vi "Read.vi"(0 "session in":T1[](array[typedef]) {"rx baseband session"."3630 session"."Address Space" items=["VXI/VME A16"=1, "VXI/VME A24"=2, "VXI/VME A32"=3, "VXI/VME A64"=4, "PXI Memory Allocations"=9, "PXI Configuration"=10, "PXI BAR0"=11, "PXI BAR1"=12, "PXI BAR2"=13, "PXI BAR3"=14, "PXI BAR4"=15, "PXI BAR5"=16]; "tx baseband session"."3610 session"."Address Space" items=["VXI/VME A16"=1, "VXI/VME A24"=2, "VXI/VME A32"=3, "VXI/VME A64"=4, "PXI Memory Allocations"=9, "PXI Configuration"=10, "PXI BAR0"=11, "PXI BAR1"=12, "PXI BAR2"=13, "PXI BAR3"=14, "PXI BAR4"=15, "PXI BAR5"=16]}, 7 "number of samples":u32=8192, 9 "master device index":i32, 11 "error in":errorcluster, 12 "Timeout (ms)":i32=5000) -> (4 "session out":T1[](array[typedef]) {"rx baseband session"."3630 session"."Address Space" items=["VXI/VME A16"=1, "VXI/VME A24"=2, "VXI/VME A32"=3, "VXI/VME A64"=4, "PXI Memory Allocations"=9, "PXI Configuration"=10, "PXI BAR0"=11, "PXI BAR1"=12, "PXI BAR2"=13, "PXI BAR3"=14, "PXI BAR4"=15, "PXI BAR5"=16]; "tx baseband session"."3610 session"."Address Space" items=["VXI/VME A16"=1, "VXI/VME A24"=2, "VXI/VME A32"=3, "VXI/VME A64"=4, "PXI Memory Allocations"=9, "PXI Configuration"=10, "PXI BAR0"=11, "PXI BAR1"=12, "PXI BAR2"=13, "PXI BAR3"=14, "PXI BAR4"=15, "PXI BAR5"=16]}, 8 "data [channel]":cluster{"data":cdb[]}[](array[cluster]), 15 "error out":errorcluster)   [LabVIEW 2019, in "mmWave HW Control.lvlib"]
uses:
  mmWave HW Control.lvlib
  Low-level/TypeDefs/Session.ctl
  <instrlib>/niMmWave/ni3620/Config/v1/Host/Public/High-Level/niMmWave Session.ctl
  <instrlib>/_niInstr/Register Bus/v0/Host/Public/Register Bus Session.ctl
  <instrlib>/_niInstr/Register Bus/v0/Host/Private/Session Data.ctl
  <instrlib>/niMmWave/ni3620/Config/v1/Host/Public/Typedefs/Board Information.ctl
  <instrlib>/niMmWave/ni3620/Config/v1/Host/Public/Typedefs/Hardware Revision.ctl
  <instrlib>/niMmWave/ni3620/Config/v1/Host/Public/Typedefs/Gain Mapping.ctl
  <instrlib>/niMmWave/ni3620/Config/v1/Host/Public/Typedefs/Correction Data.ctl
  <instrlib>/niMmWave/ni3620/Config/v1/Host/Public/Typedefs/Opera Characterization.ctl
  <instrlib>/niMmWave/ni3620/Config/v1/Host/Public/Corrections/Typedefs/Opera Characterization Main Header.ctl
  <instrlib>/niMmWave/ni3620/Config/v1/Host/Public/Corrections/Typedefs/Opera IF Board Information.ctl
  <instrlib>/niMmWave/ni3620/Config/v1/Host/Public/Corrections/Typedefs/Opera Characterization Instance Header.ctl
  <instrlib>/niMmWave/ni3620/Config/v1/Host/Public/Corrections/Typedefs/Opera Characterization Device Data Header.ctl
  <instrlib>/niMmWave/ni3620/Config/v1/Host/Public/Corrections/Typedefs/Opera LO Characterization Data Header.ctl
  <instrlib>/niMmWave/ni3620/Config/v1/Host/Public/Corrections/Typedefs/Opera IF Board Characterization Data Header.ctl
  <instrlib>/niMmWave/ni3620/Config/v1/Host/Public/Corrections/Typedefs/Opera Characterization Device Data.ctl
  <instrlib>/niMmWave/ni3620/Config/v1/Host/Public/Corrections/Typedefs/Opera LO2 Board Characterization Data.ctl
  <instrlib>/niMmWave/ni3620/Config/v1/Host/Public/Corrections/Typedefs/Opera LO Characterization Data.ctl
  <instrlib>/niMmWave/ni3620/Config/v1/Host/Public/Corrections/Typedefs/Opera IF Board Characterization Data.ctl
  <instrlib>/niMmWave/ni3620/Config/v1/Host/Public/Corrections/Typedefs/Opera IQ Impairment Data.ctl
  <instrlib>/niMmWave/ni3620/Config/v1/Host/Public/Typedefs/mmWave Adapter Session Data.ctl
  <instrlib>/niMmWave/ni3620/Config/v1/Host/Public/Typedefs/mmWave Adapter Data.ctl
  <instrlib>/niMmWave/ni3620/Config/v1/Host/Public/Typedefs/mmWave Adapter 2.ctl
  <instrlib>/niMmWave/ni3620/Config/v1/Shared/Typedefs/Subsystem ID.ctl
  <instrlib>/niMmWave/ni3620/Config/v1/Host/Public/Typedefs/mmWave Adapter Channel Information.ctl
  <instrlib>/niMmWave/ni3620/Config/v1/Host/Public/Typedefs/Temperature Coefficients.ctl
  <instrlib>/niMmWave/ni3620/Config/v1/Host/Public/Typedefs/mmWave Characterization.ctl
  <instrlib>/niMmWave/ni3620/Config/v1/Host/Public/Corrections/Typedefs/mmWave Characterization Main Header.ctl
  <instrlib>/niMmWave/ni3620/Config/v1/Host/Public/Corrections/Typedefs/mmWave Characterization Instance Header.ctl
  <instrlib>/niMmWave/ni3620/Config/v1/Host/Public/Typedefs/Session Cache.ctl
  <instrlib>/niMmWave/ni3620/Config/v1/Host/Public/Typedefs/LO2 settings cache.ctl
  <instrlib>/niMmWave/ni3620/Config/v1/Host/Public/Typedefs/LO2 source.ctl
  <instrlib>/niMmWave/ni3620/Config/v1/Host/Public/Typedefs/Desired and Coerced.ctl
  <instrlib>/niMmWave/ni3620/Config/v1/Host/Public/Typedefs/Export cache.ctl
  <instrlib>/niMmWave/ni3620/Config/v1/Host/Public/Typedefs/Path cache.ctl
  <instrlib>/niMmWave/ni3620/Config/v1/Host/Public/Typedefs/Daughterboard Type.ctl
  <instrlib>/niMmWave/ni3620/Config/v1/Host/Public/Typedefs/LO1 settings cache.ctl
  <instrlib>/niMmWave/ni3620/Config/v1/Host/Public/Typedefs/LO1 Source.ctl
  <instrlib>/niMmWave/ni3620/Config/v1/Host/Public/Typedefs/mmWave export cache.ctl
  <instrlib>/niMmWave/ni3620/Config/v1/Host/Private/Board/LO2/LO2 Board Configuration Cache.ctl
  <instrlib>/niMmWave/ni3620/Config/v1/Host/Public/Typedefs/reference clock routing settings.ctl
  <instrlib>/niMmWave/ni3620/Config/v1/Host/Public/Typedefs/LO2 routing settings.ctl
  <instrlib>/niMmWave/ni3620/Config/v1/Host/Private/Board/LO1/LO1 Board Configuration Cache.ctl
  <instrlib>/niMmWave/ni3620/Config/v1/Host/Public/Typedefs/LO1 source settings.ctl
  <instrlib>/niMmWave/ni3620/Config/v1/Host/Public/Typedefs/LO1 export settings.ctl
  <instrlib>/niMmWave/ni3620/Config/v1/Host/Public/Typedefs/LO1 mmWave settings.ctl
  Low-level/TypeDefs/Tx Baseband Session.ctl
  <instrlib>/niMmWave/ni3610 and ni3630/controls/public/Main Settings.ctl
  <vilib>/Instr/_visa.llb/VISA Register Access Address Space.ctl
  <instrlib>/niMmWave/ni3610 and ni3630/controls/public/Register Adresses.ctl
  <instrlib>/niMmWave/ni3610 and ni3630/controls/public/Base Card Type.ctl
  <instrlib>/niMmWave/ni3610 and ni3630/controls/private/IQ Card Revision.ctl
  <instrlib>/niMmWave/ni3610 and ni3630/controls/public/Board Capability.ctl
  Low-level/TypeDefs/Blank FPGA Reference.ctl
  Low-level/TypeDefs/Rx Baseband Session.ctl
  Low-level/TypeDefs/Hardware Configuration.ctl
  Low-level/TypeDefs/Direction.ctl
  Low-level/TypeDefs/Gain Ranging.ctl
  Low-level/TypeDefs/PXI Trigger Bus Info.ctl
  Low-level/TypeDefs/RX driver FPGA ref.ctl
  <vilib>/rvi/errors/niLvFpgaAdjustHostInterfaceError.vi
  <vilib>/rvi/interface/common/niFpgaWaitOnOcc.vi
  <vilib>/rvi/interface/nirviReadWriteControl/nirviReadWriteControl.xnode
  <vilib>/rvi/interface/nirviMethod/nirviMethod.xnode
  <vilib>/rvi/errors/niLvFpgaMergeErrorWithErrorCode.vi
  <vilib>/FPGAPlugInAG/Dynamic/niLvFpga_ReadFifo_Dynamic.vi
  NiFpgaLv.dll
  <vilib>/rvi/interface/Simulation/niFpgaSimulationCallBeginRW.vi
  <vilib>/FPGAPlugInAG/Dynamic/niLvFpga_ConfigureFifo_Dynamic.vi
  <vilib>/FPGAPlugInAG/Dynamic/niLvFpga_StartFifo_Dynamic.vi
  <instrlib>/_niInstr/Register Bus/v0/Host/niInstr Register Bus v0 Host.lvlib
  <instrlib>/niMmWave/ni3610 and ni3630/ni3610_and_ni3630_Driver_Lib.lvlib
  <instrlib>/niMmWave/ni3620/Config/v1/Host/niMmWave Config v1 Host.lvlib
  <instrlib>/niMmWave/ni3620/Config/v1/Shared/niMmWave Config v1 Shared.lvlib
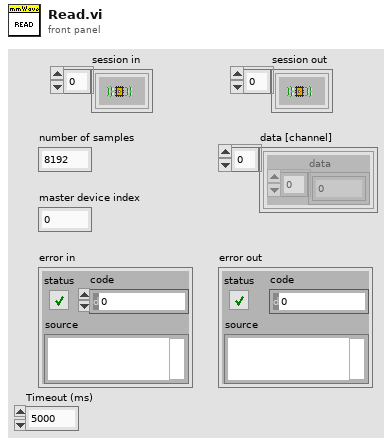
[diagram p1: front panel]
types:
  T1 = typedef "Session.ctl" = cluster{"3620 session":refnum<queue>, "tx baseband session":T2, "rx baseband session":T10, "tx gain (dB)":dbl, "rx gain (dB)":dbl, "hardware configuration":T11, "gain ranging":T13[], "pxi trigger bus information":T14}
  T2 = typedef "Tx Baseband Session.ctl" = cluster{"3610 session":T3, "7902 reference":T9}
  T3 = typedef "ni3610_and_ni3630_Driver_Lib.lvlib/Main Settings.ctl" = cluster{"VISA resource name":refnum<visa-resource-name>, "Address Space":T4, "window_offset":u32, "register_addresses":T5, "required_MM_fpga_version":cluster{"signature":u32, "hardware":u32, "current revision":u32, "oldest revision":u32}, "CPLD Oldest Compat Version ":cluster{"hardware":u32, "CPLD firmware":u32}, "MM_FPGA_image_location":string, "is_init":bool, "card_type":T6, "DacLmkConfigFileName":string, "AdcLmkConfigFileName":string, "AdcConfigFileName":string, "DacConfigFileName_RevA":string, "DacConfigFileName_RevB":string, "Mulde hardware revision":u8, "bypass DAC PLL\n":bool, "IQ Card Revision":T7, "board capability":T8}
  T4 = typedef "VISA Register Access Address Space.ctl" = u16
  T5 = typedef "ni3610_and_ni3630_Driver_Lib.lvlib/Register Adresses.ctl" = cluster{"MM based Registers":cluster{"Revision":u32, "OldestCompatRev":u32, "signature":u32, "scratch":u32, "LedControl":u32, "BoardHwRev":u32, "BoardControl":u32, "ThermalStatus":u32, "BasebandStatus":u32, "BasebandControl":u32, "BasebandAuxSetup":u32, "BasebandAuxStatus":u32, "LmkSyncOutSetup":u32, " AdcSyncOutSetup":u32, " InjSyncOutSetup":u32, " PxiTrig0OutSetup":u32, " PxiTrig1OutSetup":u32, " PxiTrig2OutSetup":u32, " PxiTrig3OutSetup":u32, " PxiTrig4OutSetup":u32, " PxiTrig5OutSetup":u32, " PxiTrig6OutSetup":u32, " PxiTrig7OutSetup":u32}, "CPLD based Registers":cluster{"SlaveSignature":u32, "SlaveRevision":u32, "SlaveOldestCompatRev":u32, "SlaveScratch":u32, "SlaveSetup":u32, "SlaveStatus":u32, "IDacReg_offset":u32, "LMKRegGrp0_offset":u32, "QDacReg_offset":u32, "BrdTempSensorVal":u32, "TempSensorPowerDown":u32, "GPIOReg_offset":u32, "IAdcReg_offset":u32, "QAdcReg_offset":u32, "LMKRegGrp1_offset":u32, "QadcTempSensorVal":u32, "IadcTempSensorVal":u32, "RevisionReg":u32, "VcxoReg":u32, "CpldStatusReg":u32, "PowerReg":u32, "VBiasEnReg":u32, "ExtRefOeReg":u32, "QdacCtrlReg":u32, "QdacStatusReg":u32, "IdacCtrlReg":u32, "IdacStatusReg":u32, "QdacJtagIn":u32, "QdacJtagOut":u32, "IdacJtagIn":u32, "IdacJtagOut":u32, "IqDcSetupReg":u32, "QadcStatusReg":u32, "IadcStatusReg":u32, "BrdSetupReg":u32, "IqDcRevisionReg":u32, "PllStatusReg":u32, "EndpointScratchReg":u32, "AdcSyncCfgReg":u32, "IqCardOpampReg":u32}, "CPLD Register Offset":u32, "MM  Register Offset":u32, " PxiTrig0OutSetup":u32}
  T6 = typedef "ni3610_and_ni3630_Driver_Lib.lvlib/Base Card Type.ctl" = enum16{"unspecified", "ADC", "DAC"}
  T7 = typedef "ni3610_and_ni3630_Driver_Lib.lvlib/IQ Card Revision.ctl" = enum16{"RevA", "RevB", "RevC", "RevD"}
  T8 = typedef "ni3610_and_ni3630_Driver_Lib.lvlib/Board Capability.ctl" = cluster{"baseband sync":enum16{"no baseband sync", "baseband sync"}}
  T9 = typedef "Blank FPGA Reference.ctl" = refnum<k20>
  T10 = typedef "Rx Baseband Session.ctl" = cluster{"3630 session":T3, "7902 reference":T9}
  T11 = typedef "Hardware Configuration.ctl" = cluster{"direction":T12, "baseband only":bool}
  T12 = typedef "Direction.ctl" = enum16{"Transceiver", "Receiver", "Transmitter"}
  T13 = typedef "Gain Ranging.ctl" = cluster{"gain ranging active scope":string, "gain ranging stream session":refnum<k20>}
  T14 = typedef "PXI Trigger Bus Info.ctl" = cluster{"chassis resource name":refnum<visa-resource-name>, "7902R (TX)":i16, "3610 (TX)":i16, "3620 (IF)":i16, "3630 (RX)":i16, "7902R (RX)":i16}
  T15 = typedef "RX driver FPGA ref.ctl" = refnum<k20>
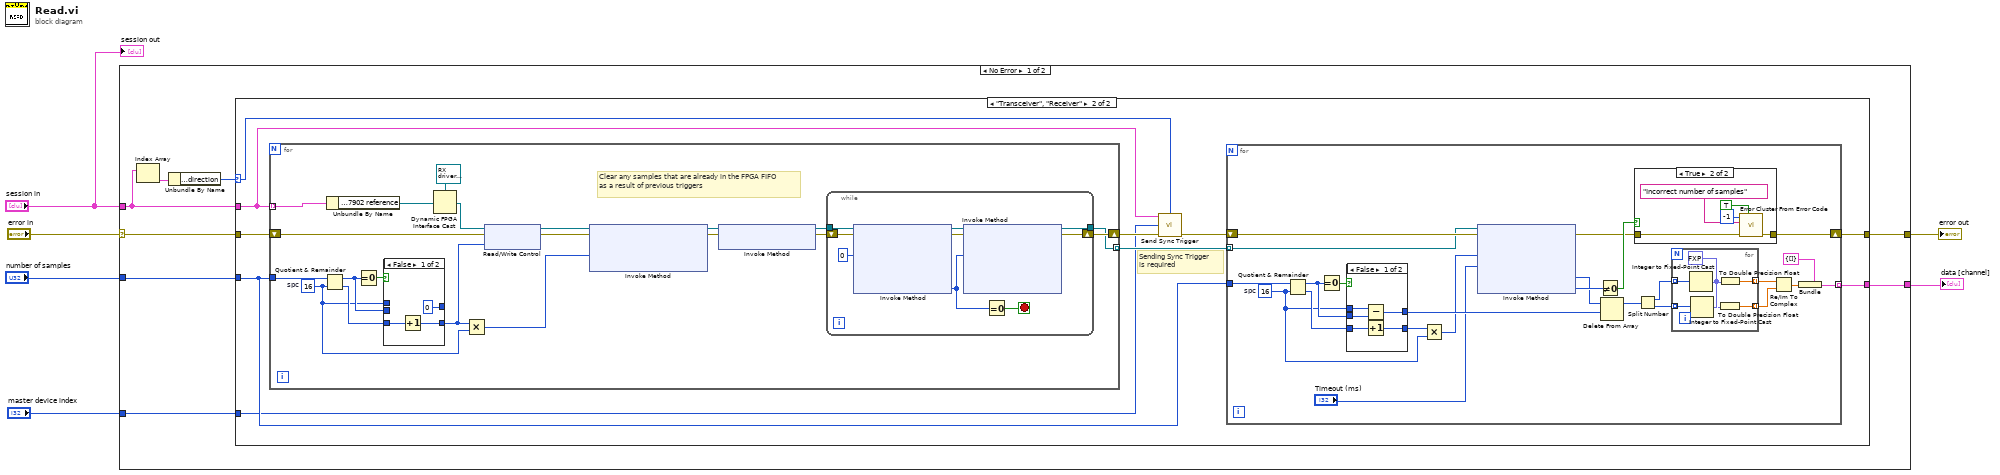
[diagram p0: block diagram]
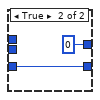
[diagram p4: hidden frame]
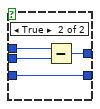
[diagram p5: hidden frame]
diagram:
  n1 = case shown="No Error" "error in" {
    selector: "error in" -> [w14 w106]
    tunnel: [w11 w106] -> w5
    tunnel: "master device index" -> [w13 _]
    tunnel: "session in" -> [w9 _]
    tunnel: "number of samples" -> [w12 _]
    tunnel: [w10 _] -> w1
    frame No Error {
      n2 = Index Array(array=w9) -> (element=w8:T1)  [unwired: 1 in]
      n3 = Unbundle By Name(w8) -> ("hardware configuration.direction"=w7:T12)
      n4 = case shown="\"Transceiver\", \"Receiver\"" w7 {
        selector: w7 -> [_ w17]
        tunnel: w14 -> [w15 w25]
        tunnel: w9 -> [_ w24]
        tunnel: w13 -> [_ w16]
        tunnel: w12 -> [_ w23]
        tunnel: [w15 w22] -> w11
        tunnel: [_ w21] -> w10
        frame "Transmitter" {
        }
        frame "Transceiver", "Receiver" {
          # "Sending Sync Trigger\nis required"
          n5 = for {
            tunnel: w24 -> [w76] mode=indexing
            tunnel: w23 -> [w74]
            shift-right: [w73] -> w20
            shift-left: w25 -> [w72]
            tunnel: [w71] -> w18 mode=indexing
            w81 = u32 16  # spc
            # "Clear any samples that are already in the FPGA FIFO\nas a result of previous triggers"
            n6 = Quotient & Remainder(x=w74, y=w81) -> (x-y*floor(x/y)=w82:u32, floor(x/y)=w83:u32)
            n7 = Unbundle By Name(w76) -> ("rx baseband session.7902 reference"=w75:T9)
            n8 = Equal To 0?(x=w82) -> (x = 0?=w84:bool)
            n9 = case shown="False" w84 {
              tunnel: w83 -> [w101 w105]
              tunnel: w82 -> [_ w104]
              tunnel: [w100 w105] -> w77
              tunnel: w81 -> [_ w103]
              tunnel: [u64 0 w102] -> _
              frame False {
                n10 = Increment(x=w101) -> (x+1=w100:u32)
              }
              frame True {
                n11 = Subtract(x=w103, y=w104) -> (x-y=w102:u32)
              }
            }
            n12 = Dynamic FPGA Interface Cast(Session In=T15 refnum ("Type"), Type=w75) -> (Session Out=w85:T15)
            n13 = Multiply(x=w77, y=w81) -> (x*y=w80:u32)
            n14 = xnode "Read/Write Control"("FPGA VI Reference In"=w85, "error in"=w72, "acq.length"=w77) -> ("FPGA VI Reference Out"=w89:T15, "error out"=w88:errorcluster)
            n15 = xnode "Invoke Method"("FPGA VI Reference In"=w89, "error in"=w88, "Requested Depth"=w80) -> ("FPGA VI Reference Out"=w87:T15, "error out"=w86:errorcluster)  [unwired: 1 out]
            n16 = xnode "Invoke Method"("FPGA VI Reference In"=w87, "error in"=w86) -> ("FPGA VI Reference Out"=w79:T15, "error out"=w78:errorcluster)
            n17 = while {
              tunnel: w79 -> [w97]
              shift-right: [w93] -> w73
              shift-left: w78 -> [w94]
              tunnel: [w91] -> w71
              stop <- w92 stop-if-true
              n18 = xnode "Invoke Method"("FPGA VI Reference In"=w97, "error in"=w94, "Number of Elements"=u32 0) -> ("FPGA VI Reference Out"=w95:T15, "error out"=w96:errorcluster, "Elements Remaining"=w90:u32)  [unwired: 1 in, 1 out]
              n19 = xnode "Invoke Method"("FPGA VI Reference In"=w95, "error in"=w96, "Number of Elements"=w90) -> ("FPGA VI Reference Out"=w91:T15, "error out"=w93:errorcluster)  [unwired: 1 in, 2 out]
              n20 = Equal To 0?(x=w90) -> (x = 0?=w92:bool)
            }
          }
          n21 = call "Send Sync Trigger.vi"("session in"=w24, "sync select"=w17, "master device index"=w16, "error in"=w20) -> ("error out"=w19:errorcluster)  [unwired: 10 in, 1 out]
          n22 = for {
            tunnel: w18 -> [w27] mode=indexing
            tunnel: w23 -> [w48]
            shift-right: [w31] -> w22
            shift-left: w19 -> [w49]
            tunnel: [w28] -> w21 mode=indexing
            w41 = u32 16  # spc
            n23 = Quotient & Remainder(x=w48, y=w41) -> (x-y*floor(x/y)=w43:u32, floor(x/y)=w44:u32)
            n24 = Equal To 0?(x=w43) -> (x = 0?=w45:bool)
            n25 = case shown="False" w45 {
              tunnel: w44 -> [w67 w69]
              tunnel: w43 -> [w65 _]
              tunnel: [w66 w69] -> w42
              tunnel: w41 -> [w64 _]
              tunnel: [w63 u64 0] -> w40
              frame False {
                n26 = Subtract(x=w64, y=w65) -> (x-y=w63:u32)
                n27 = Increment(x=w67) -> (x+1=w66:u32)
              }
              frame True {
              }
            }
            n28 = Multiply(x=w42, y=w41) -> (x*y=w34:u32)
            n29 = xnode "Invoke Method"("FPGA VI Reference In"=w27, "error in"=w49, "Number of Elements"=w34, "Timeout (ms)"="Timeout (ms)") -> ("error out"=w32:errorcluster, "Data"=w46:u32[], "Elements Remaining"=w47:u32)  [unwired: 1 out]
            n30 = Not Equal To 0?(x=w47) -> (x != 0?=w33:bool)
            n31 = Delete From Array(array=w46, length=w40) -> (array with subset deleted=w35:u32[])  [unwired: 1 in, 1 out]
            n32 = case shown="True" w33 {
              tunnel: w32 -> [w50 w55]
              tunnel: [w50 w54] -> w31
              frame False {
              }
              frame True {
                n33 = call <vilib>:"Error Cluster From Error Code.vi"("show call chain? (False)"=TRUE, "error in (no error)"=w55, "error message (\"\")"="Incorrect number of samples" ("source"), "error code (0)"=-1) -> ("error out"=w54:errorcluster)  [unwired: 5 in]
              }
            }
            n34 = Split Number(x=w35) -> (hi(x)=w39:u16[], lo(x)=w38:u16[])
            n35 = for {
              tunnel: w39 -> [w62] mode=indexing
              tunnel: w38 -> [w61] mode=indexing
              tunnel: [w57] -> w36 mode=indexing
              tunnel: [w56] -> w37 mode=indexing
              w60 = fxp<+/-,16,1> 0.0 ("fixed-point type")
              n36 = Integer to Fixed-Point Cast(fixed-point type=w60, integer=w62) -> (fixed-point=w59:fxp<+/-,16,1>)
              n37 = Integer to Fixed-Point Cast(fixed-point type=w60, integer=w61) -> (fixed-point=w58:fxp<+/-,16,1>)
              n38 = To Double Precision Float(number=w58) -> (double precision float=w56:dbl)
              n39 = To Double Precision Float(number=w59) -> (double precision float=w57:dbl)
            }
            n40 = Re/Im To Complex(1:w37, 2:w36) -> (0:w30:cdb[])
            n41 = Bundle(cluster=cluster{"data":cdb[]} {"data"=[]} ("data"), "data"=w30) -> (w28:cluster{"data":cdb[]})
          }
        }
      }
    }
    frame Error {
    }
  }
  "error out" <- w5
  "data [channel]" <- w1
  "session out" <- "session in"
